vi "Splash Screen Template.vi"() -> ()   [LabVIEW 2016, in "SLL Splash Screen.lvlib"]
uses:
  SLL Splash Screen.lvlib
panel:
  out "Splash Screen Status":string
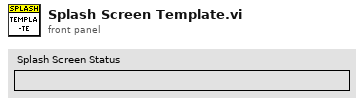
[diagram p1: front panel]
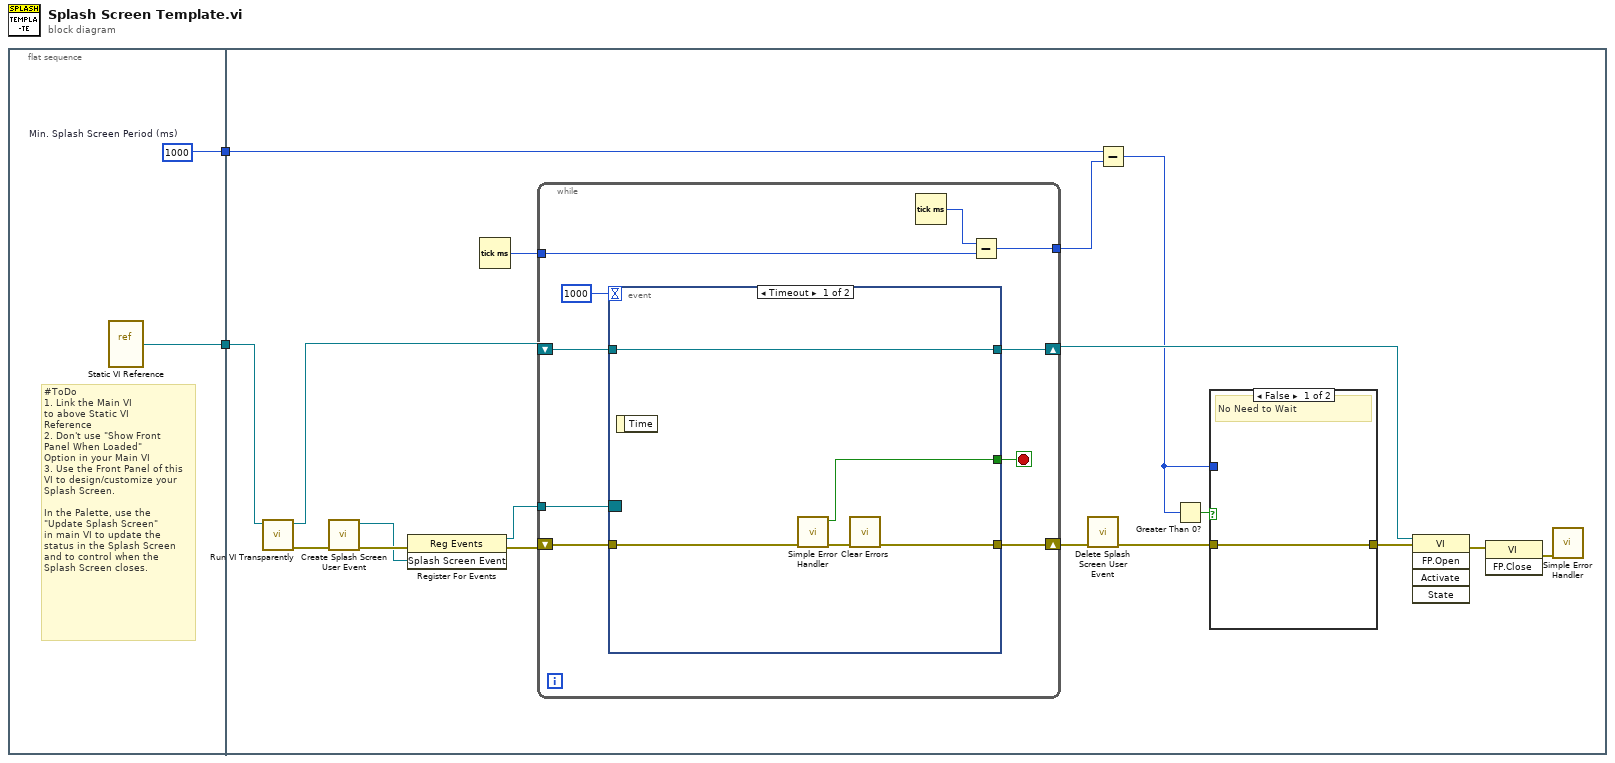
[diagram p0: block diagram]
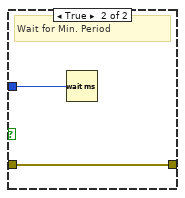
[diagram p2: hidden frame]
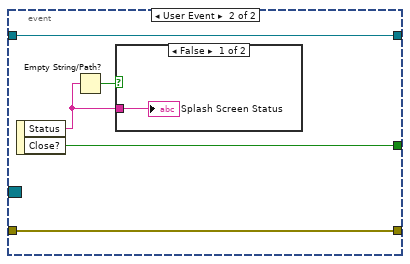
[diagram p3: hidden frame]
diagram:
  n1 = flat-sequence {
    tunnel: [w3] -> w2
    tunnel: [w4] -> w1
    tunnel: w2 -> [w6]
    tunnel: w1 -> [w15]
    frame #0 {
      w4 = u32 1000  # Min. Splash Screen Period (ms)
      # "#ToDo\n1. Link the Main VI\nto above Static VI\nReference\n2. Don't use \"Show Front\nPanel When Loaded\"\nOption in your Main VI\n3. Use the Front Panel of this\nVI to design/customize your\nSplash Screen.\n\nIn the Palette, use the \n\"Update Splash Screen\"\nin main VI to update the\nstatus in the Splash Screen\nand to control when the\nSplash Screen closes."
      n2 = vi-ref "Static VI Reference"() -> ("vi reference"=w3:refnum<vi>)
    }
    frame #1 {
      n3 = call "Run VI Transparently.vi"("VI Ref In"=w6) -> ("error out"=w7:errorcluster, "VI Ref Out"=w5:refnum<vi>)  [unwired: 9 in]
      n4 = call "Create Splash Screen User Event.vi"("error in (no error)"=w7) -> ("error out"=w20:errorcluster, "Splash Screen Event"=w18:refnum<user-event>)  [unwired: 9 in]
      n5 = register-events(error in=w20, w18) -> (reference out=w17:refnum<event-registration>, error out=w19:errorcluster)  [unwired: 1 in]
      n6 = Tick Count (ms)() -> (millisecond timer value=w16:u32)
      n7 = while {
        shift-right: [w33] -> w22
        shift-left: w5 -> [w32]
        shift-right: [w30] -> w9
        shift-left: w19 -> [w31]
        tunnel: w17 -> [w29]
        tunnel: w16 -> [w27]
        tunnel: [w26] -> w14
        stop <- w34 stop-if-true
        n8 = event shown="[0] Timeout" {
          selector: w29 -> [_ _]
          dyn-events: _ -> [_ _]
          timeout: 1000 -> [_ _]
          tunnel: [w37 w43] -> w34
          tunnel: [w40 w45] -> w33
          tunnel: w32 -> [w40 w45]
          tunnel: w31 -> [w39 w44]
          tunnel: [w36 w44] -> w30
          event Timeout {
            n9 = event-data() -> ()  [unwired: 1 in, 1 out]
            n10 = call <vilib>:"Simple Error Handler.vi"("error in (no error)"=w39) -> ("error?"=w37:bool, "error out"=w38:errorcluster)  [unwired: 4 in, 3 out]
            n11 = call <vilib>:"Clear Errors.vi"("error in (no error)"=w38) -> ("error out"=w36:errorcluster)  [unwired: 5 in, 1 out]
          }
          event User Event {
            n12 = event-data() -> ("Status"=w41:string, "Close?"=w43:bool)  [unwired: 1 in]
            n13 = Empty String/Path?(string/path=w41) -> (empty?=w42:bool)
            n14 = case shown="False" w42 {
              tunnel: w41 -> [w46 _]
              frame False {
                "Splash Screen Status" <- w46
              }
              frame True {
              }
            }
          }
        }
        n15 = Tick Count (ms)() -> (millisecond timer value=w28:u32)
        n16 = Subtract(x=w28, y=w27) -> (x-y=w26:u32)
      }
      n17 = call "Delete Splash Screen User Event.vi"("error in (no error)"=w9) -> ("error out"=w8:errorcluster)  [unwired: 10 in]
      n18 = Subtract(x=w15, y=w14) -> (x-y=w12:u32)
      n19 = Greater Than 0?(x=w12) -> (x > 0?=w13:bool)
      n20 = case shown="False" w13 {
        tunnel: w8 -> [w23 w24]
        tunnel: w12 -> [_ w25]
        tunnel: [w23 w24] -> w11
        frame False {
          # "No Need to Wait"
        }
        frame True {
          # "Wait for Min. Period"
          n21 = Wait (ms)(milliseconds to wait=w25) -> ()  [unwired: 1 out]
        }
      }
      n22 = invoke class="VI" method="FP.Open"(reference=w22, error in=w11) -> (error out=w21:errorcluster)  [unwired: 3 in, 4 out]
      n23 = invoke class="VI" method="FP.Close"(error in=w21) -> (error out=w10:errorcluster)  [unwired: 2 in, 2 out]
      n24 = call <vilib>:"Simple Error Handler.vi"("error in (no error)"=w10) -> ()  [unwired: 4 in, 5 out]
    }
  }
